vi "Read RawData.vi"(0 "DET_BUNCH in":refnum<class "Avantes_bunch.lvclass">, 5 "# of scans":i32, 9 "repump_max_value":bool, 11 "error in (no error)":errorcluster) -> (3 "first elyse clock count":dbl, 4 "DET_BUNCH out":refnum<class "Avantes_bunch.lvclass">, 6 "Channel I":sgl[][](array[numeric]), 8 "WCM_values":T1, 10 "Channel II":sgl[][](array[numeric]), 15 "error out":errorcluster)   [LabVIEW 2020, in "Avantes_bunch.lvclass"]
uses:
  Avantes_bunch.lvclass
  def_repump_values_array.ctl
  Oscilloscope/def_repump_value.ctl
  Avantes_bunch.lvclass/Avantes_bunch.ctl
  Detector.lvclass
panel:
  in  "Vizualize":bool
  out "Graphe 2":sgl[](graph)
  out "Graphe":sgl[](graph)
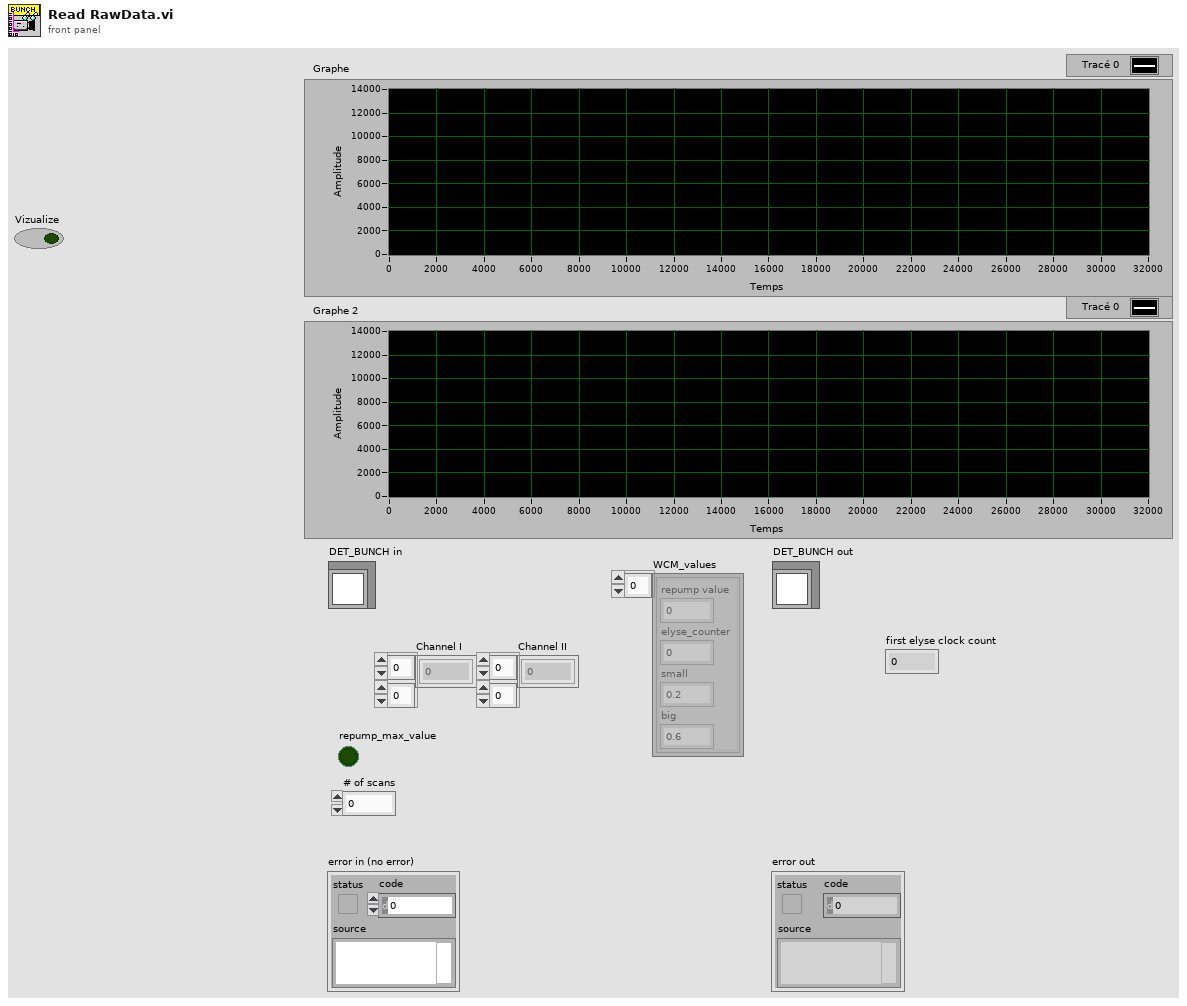
[diagram p1: front panel]
types:
  T1 = typedef "def_repump_values_array.ctl" = T2[]
  T2 = typedef "def_repump_value.ctl" = cluster{"repump value":dbl, "elyse_counter":i64, "small":dbl, "big ":dbl}
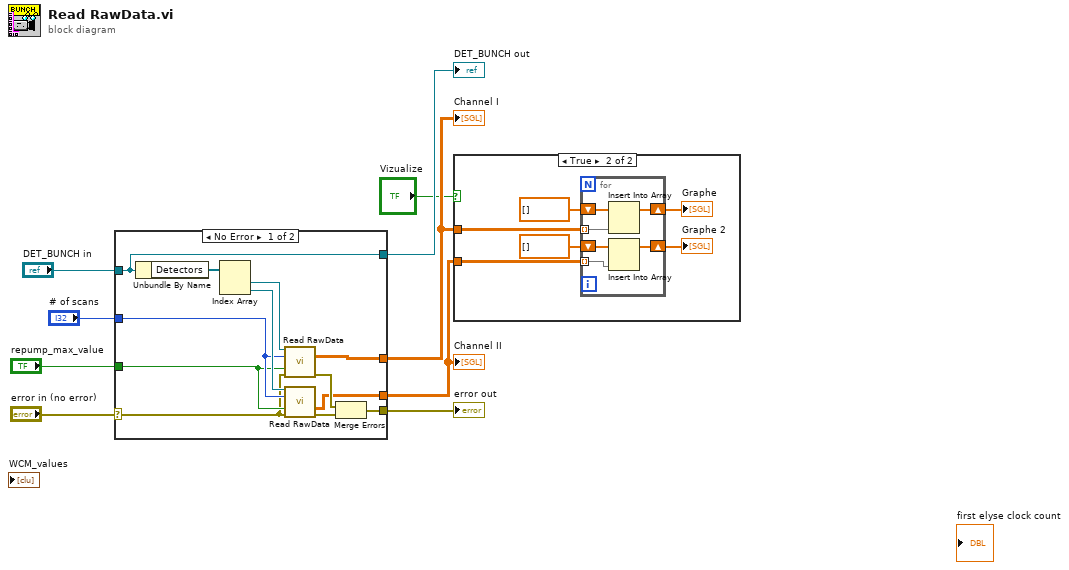
[diagram p0: block diagram]
diagram:
  n1 = case shown="No Error" "error in (no error)" {
    selector: "error in (no error)" -> [w16 w23]
    tunnel: [w13 w23] -> w8
    tunnel: [w12 w22] -> w7
    tunnel: "DET_BUNCH in" -> [w12 w22]
    tunnel: "# of scans" -> [w18 _]
    tunnel: "repump_max_value" -> [w17 _]
    tunnel: [w11 _] -> w3
    tunnel: [w10 _] -> w2
    frame No Error {
      n2 = Unbundle By Name(w12) -> ("Detectors"=w21:refnum<class "Detector.lvclass">[])
      n3 = Index Array(array=w21) -> (element #1=w20:refnum<class "Detector.lvclass">, element #2=w19:refnum<class "Detector.lvclass">)  [unwired: 2 in]
      n4 = call-dynamic "Read RawData.vi"("Detector in"=w20, "# of scans"=w18, "repump"=w17, "error in (no error)"=w16) -> ("Channel I"=w11:sgl[][], "error out"=w15:errorcluster)  [unwired: 6 in, 4 out]
      n5 = call-dynamic "Read RawData.vi"("Detector in"=w19, "# of scans"=w18, "repump"=w17, "error in (no error)"=w16) -> ("Channel II"=w10:sgl[][], "error out"=w14:errorcluster)  [unwired: 6 in, 4 out]
      n6 = Merge Errors(w15, w14) -> (w13:errorcluster)
    }
    frame Error {
    }
  }
  "error out" <- w8
  "DET_BUNCH out" <- w7
  "Channel II" <- w2
  "Channel I" <- w3
  n7 = case shown="True" "Vizualize" {
    tunnel: w3 -> [_ w28]
    tunnel: w2 -> [_ w25]
    frame False {
    }
    frame True {
      n8 = for {
        tunnel: w28 -> [w33] mode=indexing
        shift-right: [w34] -> w27
        shift-left: sgl[] [] ("Channel I") -> [w35]
        shift-right: [w31] -> w24
        shift-left: sgl[] [] ("Channel I") -> [w32]
        tunnel: w25 -> [w30] mode=indexing
        n9 = Insert Into Array(array=w35, new element=w33) -> (w34:sgl[])  [unwired: 1 in]
        n10 = Insert Into Array(array=w32, new element=w30) -> (w31:sgl[])  [unwired: 1 in]
      }
      "Graphe" <- w27
      "Graphe 2" <- w24
    }
  }
